vi "History remove zeros.vi"(3 "History XY In":T2(array[cluster])) -> (1 "History XY Out":T1(array[cluster]))   [LabVIEW 2013]
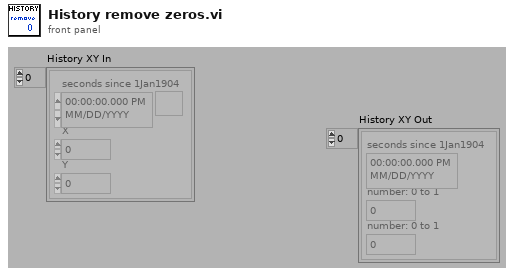
[diagram p1: front panel]
types:
  T1 = cluster{"seconds since 1Jan1904":timestamp, "number: 0 to 1":dbl, "number: 0 to 1":dbl}[]
  T2 = cluster{"seconds since 1Jan1904":timestamp, "X":dbl, "Y":dbl}[]
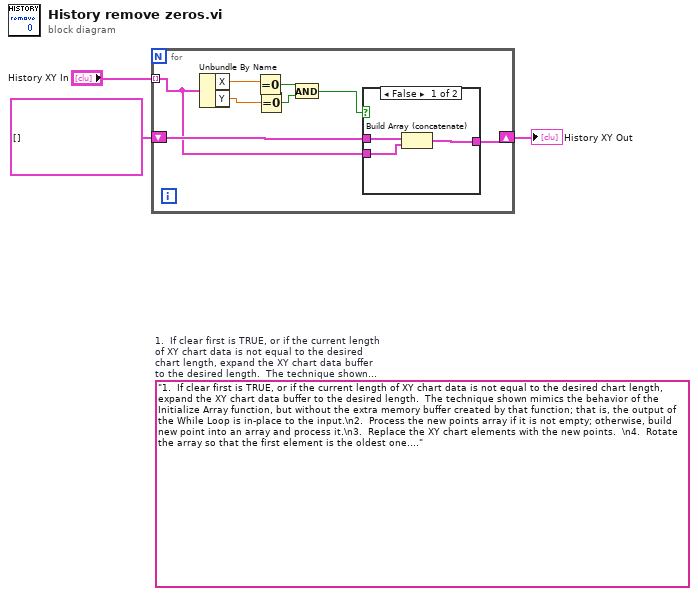
[diagram p0: block diagram]
diagram:
  (unwired) "1.  If clear first is TRUE, or if the current length of XY chart data is not equal to the desired chart length, expand the XY chart data buffer to the desired length.  The technique shown mimics the behavior of the Initialize Array function, but without the extra memory buffer created by that function; that is, the output of the While Loop is in-place to the input.\n2.  Process the new points array if it is not empty; otherwise, build new point into an array and process it.\n3.  Replace the XY chart elements with the new points.  \n4.  Rotate the array so that the first element is the oldest one.\nb marks a diagram array buffer; b? marks a buffer that may be in the calling VI. "  # 1.  If clear first is TRUE, or if the current length of XY chart data is not equal to the desired chart length, expand the XY chart data buffer to the desired length.  The technique shown mimics the behavior of the Initialize Array function, but without the extra memory buffer created by that function; that is, the output of the While Loop is in-place to the input. 2.  Process the new points array if it is not empty; otherwise, build new point into an array and process it. 3.  Replace the XY chart elements with the new points.   4.  Rotate the array so that the first element is the oldest one. b marks a diagram array buffer; b? marks a buffer that may be in the calling VI.
  n1 = for {
    tunnel: "History XY In" -> [w4] mode=indexing
    shift-right: [w6] -> w2
    shift-left: T2 [] -> [w7]
    n2 = Unbundle By Name(w4) -> ("X"=w11:dbl, "Y"=w10:dbl)
    n3 = Equal To 0?(x=w11) -> (x = 0?=w9:bool)
    n4 = Equal To 0?(x=w10) -> (x = 0?=w8:bool)
    n5 = And(x=w9, y=w8) -> (x .and. y?=w5:bool)
    n6 = case shown="False" w5 {
      tunnel: w7 -> [w14 w15]
      tunnel: [w13 w15] -> w6
      tunnel: w4 -> [w12 _]
      frame False {
        n7 = Build Array (concatenate)(w14, w12) -> (w13:T2)
      }
      frame True {
      }
    }
  }
  "History XY Out" <- w2
